vi "PVAL_get.vi"(6 "zeros(P,1)":dbl[](array[numeric]), 7 "dfe":i32, 9 "SE":dbl[](array[numeric]), 10 "B":dbl[](array[numeric]), 11 "In":dbl[](array[numeric])) -> (3 "PVAL":dbl[](array[numeric]))   [LabVIEW 2014]
uses:
  <vilib>/gmath/statdist.llb/Student t CDF.vi
  <vilib>/gmath/NI_Gmath.lvlib
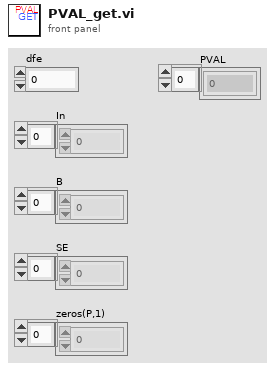
[diagram p1: front panel]
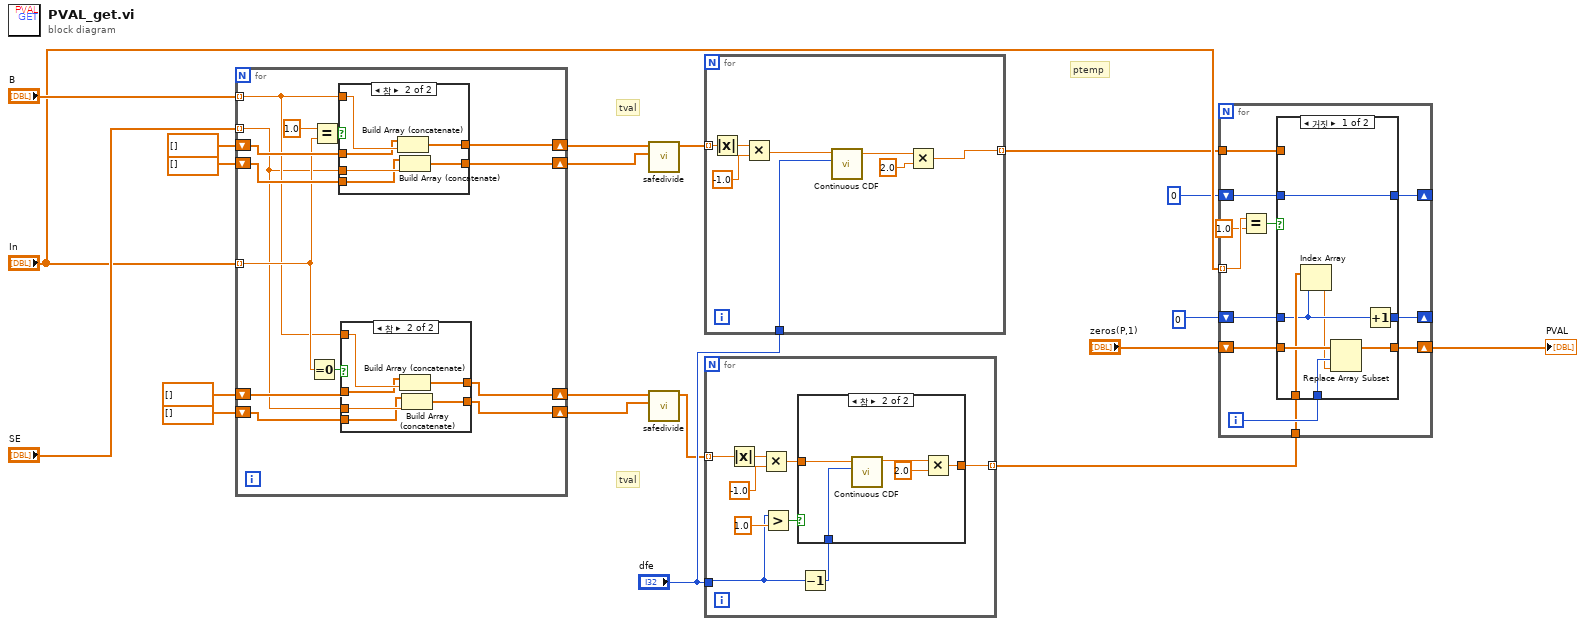
[diagram p0: block diagram]
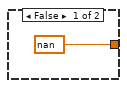
[diagram p2: hidden frame]
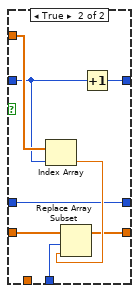
[diagram p3: hidden frame]
diagram:
  # "tval"
  # "ptemp"
  # "tval"
  n1 = for {
    tunnel: "B" -> [w22] mode=indexing
    tunnel: "SE" -> [w21] mode=indexing
    tunnel: "In" -> [w23] mode=indexing
    shift-right: [w31] -> w8
    shift-left: dbl[] [] -> [w30]
    shift-right: [w32] -> w9
    shift-left: dbl[] [] -> [w29]
    shift-right: [w26] -> w2
    shift-left: dbl[] [] -> [w28]
    shift-right: [w25] -> w1
    shift-left: dbl[] [] -> [w27]
    n2 = Equal To 0?(x=w23) -> (x = 0?=w24:bool)
    n3 = Equal?(x=1.0, y=w23) -> (x = y?=w34:bool)
    n4 = case shown="참" w34 {
      tunnel: w22 -> [_ w50]
      tunnel: w21 -> [_ w49]
      tunnel: [w43 w48] -> w32
      tunnel: [w44 w47] -> w31
      tunnel: w30 -> [w44 w46]
      tunnel: w29 -> [w43 w45]
      frame False {
      }
      frame True {
        n5 = Build Array (concatenate)(w46, w50) -> (w47:dbl[])
        n6 = Build Array (concatenate)(w45, w49) -> (w48:dbl[])
      }
    }
    n7 = case shown="참" w24 {
      tunnel: w22 -> [_ w42]
      tunnel: w21 -> [_ w41]
      tunnel: [w35 w40] -> w25
      tunnel: [w36 w39] -> w26
      tunnel: w28 -> [w36 w38]
      tunnel: w27 -> [w35 w37]
      frame False {
      }
      frame True {
        n8 = Build Array (concatenate)(w38, w42) -> (w39:dbl[])
        n9 = Build Array (concatenate)(w37, w41) -> (w40:dbl[])
      }
    }
  }
  n10 = call "safedivide.vi"("row_vec(sum)"=w9, "V' x A"=w8) -> ("Array"=w10:dbl[])  [unwired: 9 in]
  n11 = call "safedivide.vi"("row_vec(sum)"=w1, "V' x A"=w2) -> ("Array"=w18:dbl[])  [unwired: 9 in]
  n12 = for {
    tunnel: w10 -> [w58] mode=indexing
    tunnel: [w52] -> w11 mode=indexing
    tunnel: "dfe" -> [w51]
    n13 = Absolute Value(x=w58) -> (abs(x)=w57:dbl)
    n14 = Multiply(x=w57, y=-1.0) -> (x*y=w56:dbl)
    n15 = call-poly <vilib>:"Continuous CDF.vi"("k degrees of freedom"=w51, "x"=w56) -> ("cdf(x)"=w54:dbl)  [unwired: 7 in, 2 out]
    n16 = Multiply(x=w54, y=2.0) -> (x*y=w52:dbl)
  }
  n17 = for {
    tunnel: w18 -> [w65] mode=indexing
    tunnel: [w63] -> w5 mode=indexing
    tunnel: "dfe" -> [w59]
    n18 = Absolute Value(x=w65) -> (abs(x)=w67:dbl)
    n19 = Multiply(x=w67, y=-1.0) -> (x*y=w64:dbl)
    n20 = Greater?(x=w59, y=1.0) -> (0:w61:bool)
    n21 = Decrement(x=w59) -> (x-1=w62:i32)
    n22 = case shown="참" w61 {
      tunnel: w64 -> [_ w71]
      tunnel: [nan ("element") w70] -> w63
      tunnel: w62 -> [_ w69]
      frame False {
      }
      frame True {
        n23 = call-poly <vilib>:"Continuous CDF.vi"("k degrees of freedom"=w69, "x"=w71) -> ("cdf(x)"=w73:dbl)  [unwired: 7 in, 2 out]
        n24 = Multiply(x=w73, y=2.0) -> (x*y=w70:dbl)
      }
    }
  }
  n25 = for {
    tunnel: "In" -> [w84] mode=indexing
    tunnel: w11 -> [w82]
    shift-right: [w80] -> w19
    shift-left: "zeros(P,1)" -> [w81]
    shift-right: [w77] -> _
    shift-left: 0 -> [w78]
    shift-right: [w75] -> _
    shift-left: 0 -> [w76]
    tunnel: w5 -> [w74]
    i -> [w79]
    n26 = Equal?(x=w84, y=1.0) -> (x = y?=w85:bool)
    n27 = case shown="거짓" w85 {
      tunnel: w82 -> [_ w98]
      tunnel: w81 -> [w93 w101]
      tunnel: [w91 w95] -> w80
      tunnel: w79 -> [w90 w100]
      tunnel: w78 -> [w92 w97]
      tunnel: [w92 w99] -> w77
      tunnel: w76 -> [w87 w94]
      tunnel: [w89 w94] -> w75
      tunnel: w74 -> [w88 _]
      frame False {
        n28 = Index Array(array=w88, index=w87) -> (element=w86:dbl)
        n29 = Replace Array Subset(array=w93, new element=w86, index=w90) -> (w91:dbl[])
        n30 = Increment(x=w87) -> (x+1=w89:i32)
      }
      frame True {
        n31 = Index Array(array=w98, index=w97) -> (element=w96:dbl)
        n32 = Replace Array Subset(array=w101, new element=w96, index=w100) -> (w95:dbl[])
        n33 = Increment(x=w97) -> (x+1=w99:i32)
      }
    }
  }
  "PVAL" <- w19
